vi "ReadWrite.WriteValues.vi"(8 "error in":errorcluster, 10 "Values":dbl[](array[numeric]), 11 "ReadWrite in":refnum<class "ReadWrite.lvclass">) -> (0 "error out":errorcluster, 3 "ReadWrite out":refnum<class "ReadWrite.lvclass">)   [LabVIEW 2024, in "VS Plugin Data Access Engine.lvlib" / "ReadWrite.lvclass"]
uses:
  ReadWrite.lvclass
  ReadWrite.lvclass/ReadWrite.ctl
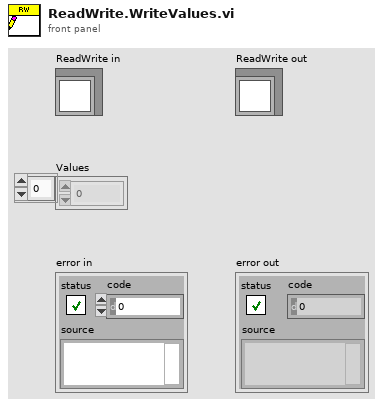
[diagram p1: front panel]
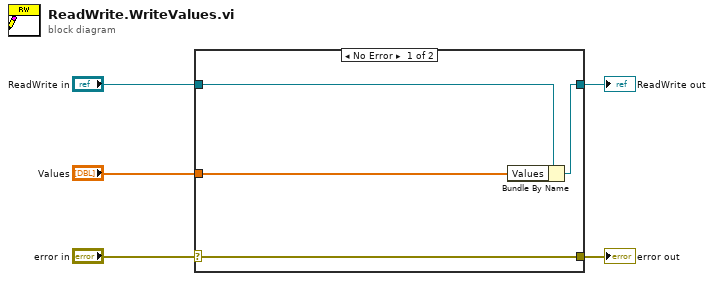
[diagram p0: block diagram]
diagram:
  n1 = case shown="No Error" "error in" {
    selector: "error in" -> [w9 w11]
    tunnel: [w9 w11] -> w4
    tunnel: [w7 w10] -> w2
    tunnel: "ReadWrite in" -> [w8 w10]
    tunnel: "Values" -> [w6 _]
    frame No Error {
      n2 = Bundle By Name(cluster=w8, "Values"=w6) -> (w7:refnum<class "ReadWrite.lvclass">)
    }
    frame Error {
    }
  }
  "error out" <- w4
  "ReadWrite out" <- w2
